vi "SPI_Example_Port Code_kyles_new_SM.vi"(11 "FPGA IO":T1={"SCLK"="DIO18", "CS_1"="DIO16", "MOSI"="DIO26", "MISO"="DIO25"}) -> ()   [LabVIEW 2012]
uses:
  Controls/FPGA SPI_Port Loop State.ctl
  <vilib>/rvi/DataTransferAndStorage/Container/Common/niFpgaContainerMetaDataKey.ctl
  <vilib>/rvi/DataTransferAndStorage/Container/Common/niFpgaContainerState.ctl
  <vilib>/rvi/DataTransferAndStorage/Container/Common/niFpgaDataTypeControl.ctl
  <vilib>/rvi/DataTransferAndStorage/Container/Common/niFpgaContainerImplementationControl.ctl
  <vilib>/rvi/DataTransferAndStorage/Container/Common/niFpgaContainerArbitrationOptionsControl.ctl
  <vilib>/rvi/DataTransferAndStorage/Container/Common/niFpgaTransferTypeControl.ctl
  <vilib>/rvi/DataTransferAndStorage/Container/Common/niFpgaContainerInitializationParameters.ctl
  <vilib>/rvi/Memory/Memory_Types/niFpgaMemoryInterfaceConfiguration.ctl
  <vilib>/rvi/FIFO/Fifo_Types/niFpgaFifoControlLogicControl.ctl
  Controls/FPGA SPI_SPI Loop State.ctl
  <vilib>/rvi/DataTransferAndStorage/Container/Common/niFpgaContainerGetUniqueNameForEmu.vi
  <vilib>/rvi/DataTransferAndStorage/Container/Common/niFpgaContainerSetEmuInfo.vi
  <vilib>/rvi/eio/common/nirviEmuReportErrorAndStop.vi
  Code/FPGA SPI_Globals.vi
  <vilib>/rvi/Emulation/niFpgaSctlEmulationGetInTimedLoop.vi
  <vilib>/rvi/Emulation/niFpgaSctlEmulationGlobalWrite.vi
  <vilib>/rvi/FIFO/Fifo_Resource/nirvififoEmulationSetSize.vi
  <vilib>/rvi/Emulation/niFpgaSctlEmulationFifoFullMgr.vi
  <vilib>/rvi/errors/niFpgaSetErrorForExecOnDevCompSimple.vi
  <vilib>/rvi/Emulation/niFpgaSctlEmulationResourceMgr.vi
  <vilib>/rvi/eio/common/nirviEmuTemplateMethod_errors.vi
  <vilib>/rvi/LocalResourceManager/LocalResourceManager.xnode
  <vilib>/rvi/DataTransferAndStorage/Container/XNode/niFpgaContainer.xnode
  <vilib>/rvi/FIFO/Fifo_Resource/nirvififoEmulationRead.vi
  <vilib>/rvi/FIFO/Fifo_Resource/nirvififoEmulationWrite.vi
  <vilib>/eio/EIONode/EIONode.xnode
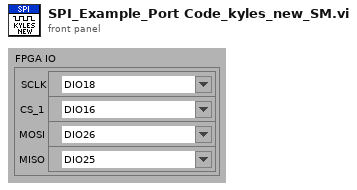
[diagram p1: front panel]
types:
  T1 = cluster{"SCLK":refnum<k21>, "CS_1":refnum<k21>, "MOSI":refnum<k21>, "MISO":refnum<k21>}
  T2 = typedef "FPGA SPI_Port Loop State.ctl" = enum8{"Idle", "Start", "Configure Hardware", "Start Hardware", "Set Done", "Wait Until Done", "Restart Port"}
  T3 = typedef "FPGA SPI_SPI Loop State.ctl" = enum8{"Initialize", "Set CS", "Read From FIFO", "Send Byte", "Write to FIFO", "Reset CS", "Read Delay"}
  T4 = typedef "FPGA SPI_Cmd.ctl" = enum8{"Idle", "Write/Read SPI", "Configure", "Restart"}
  T5 = cluster{"MOSI":bool[], "MISO":bool[], "Read?":bool}
  T6 = cluster{"Next State":T3, "Total Bytes":u16, "Future State":T3, "Read Wait":u32, "CS Reset Wait":u32, "Byte Count":u16}
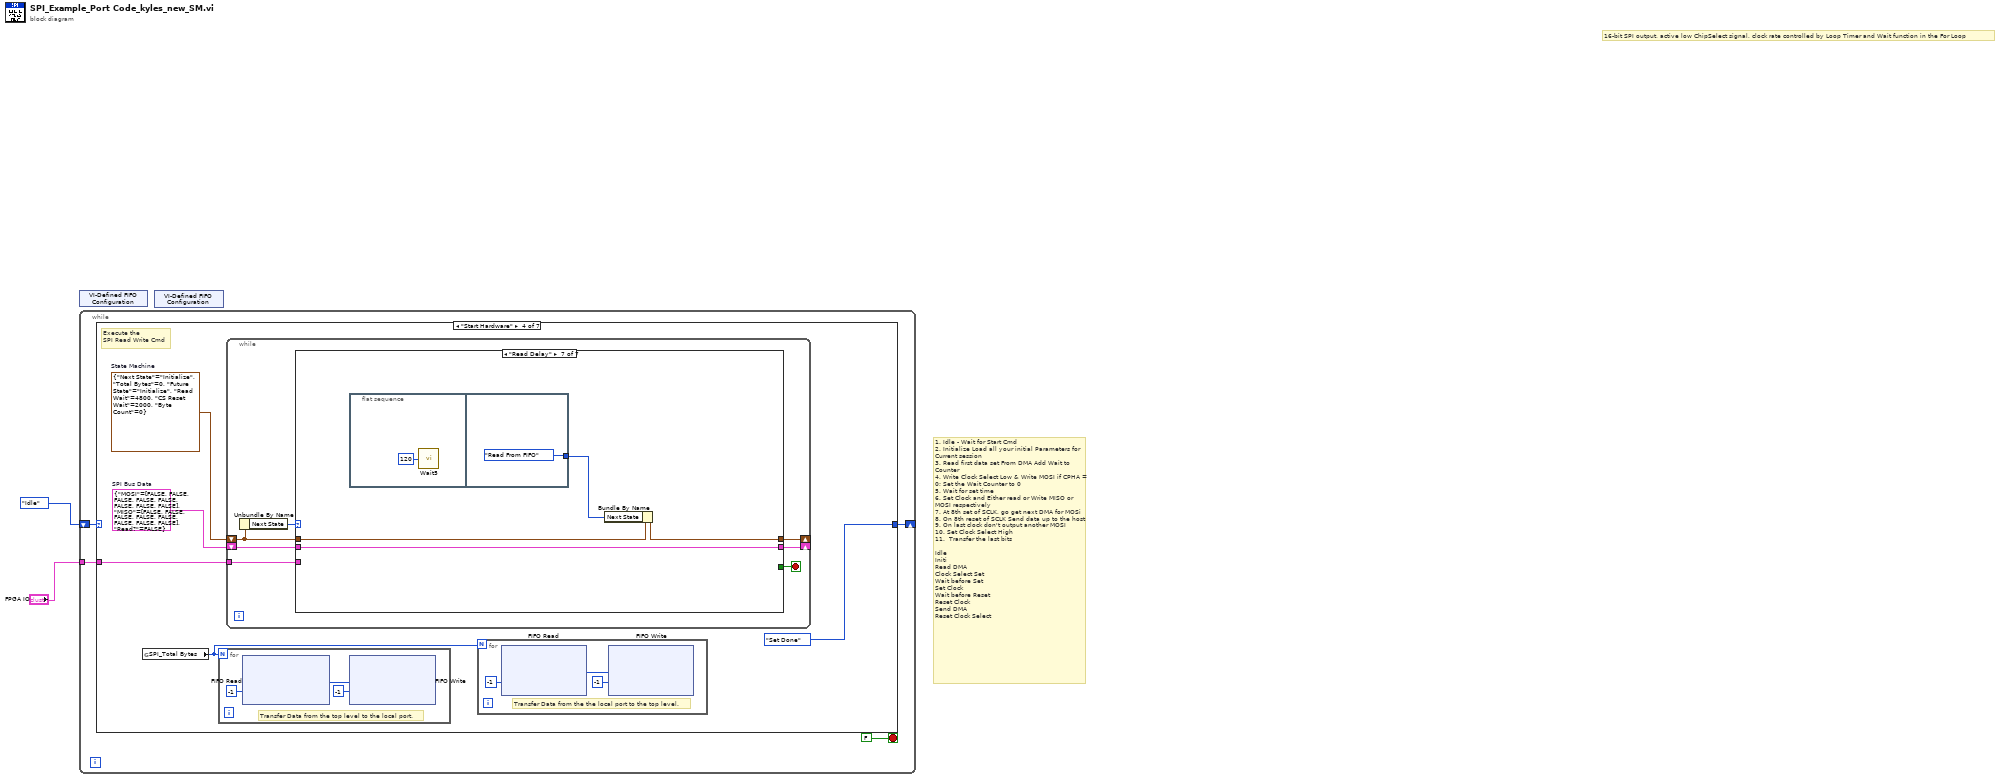
[diagram p0: block diagram]
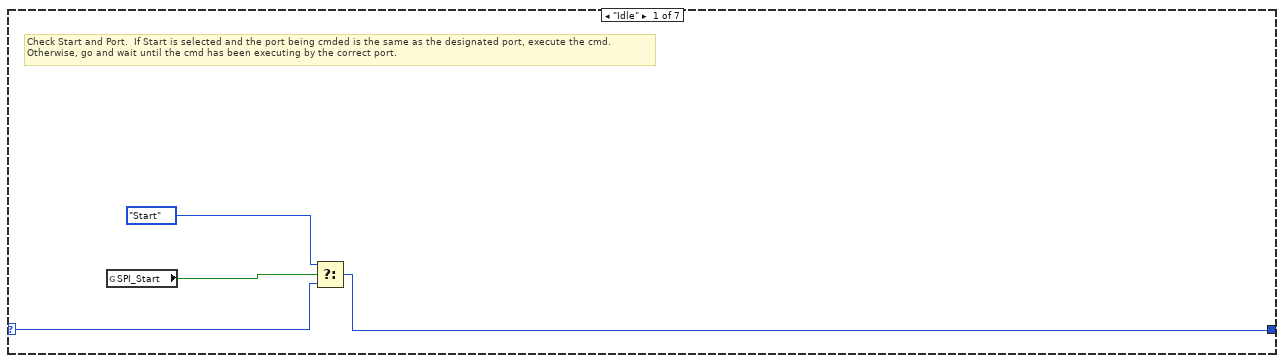
[diagram p2: hidden frame]
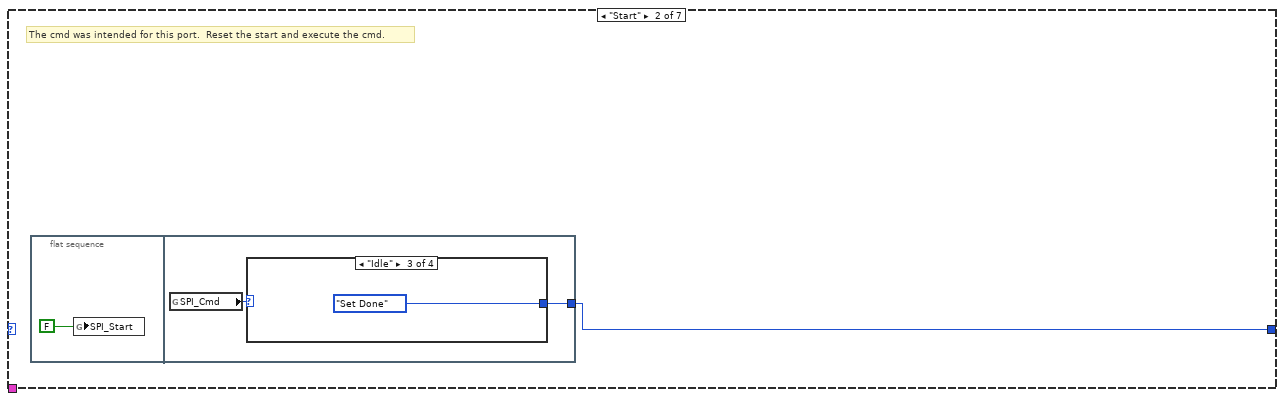
[diagram p3: hidden frame]
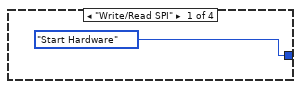
[diagram p4: hidden frame]
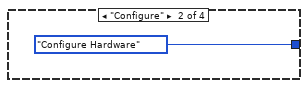
[diagram p5: hidden frame]
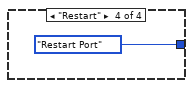
[diagram p6: hidden frame]
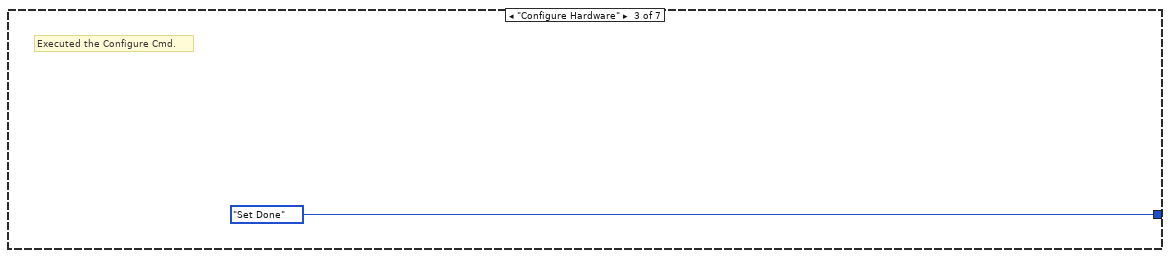
[diagram p7: hidden frame]
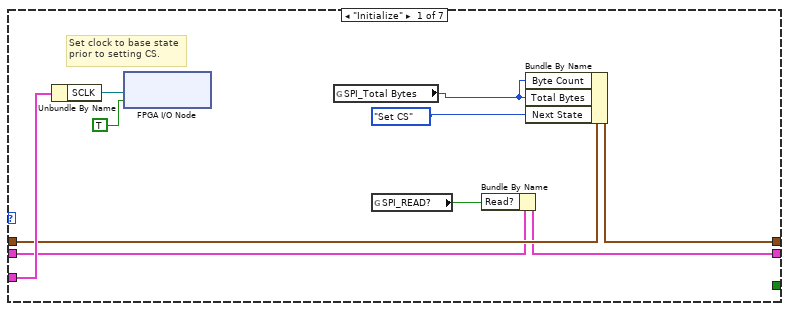
[diagram p8: hidden frame]
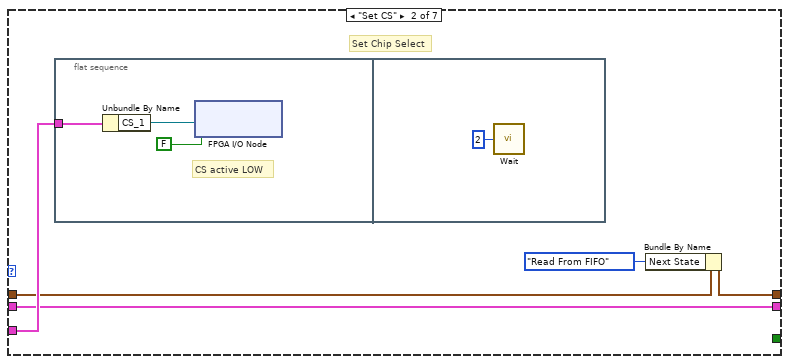
[diagram p9: hidden frame]
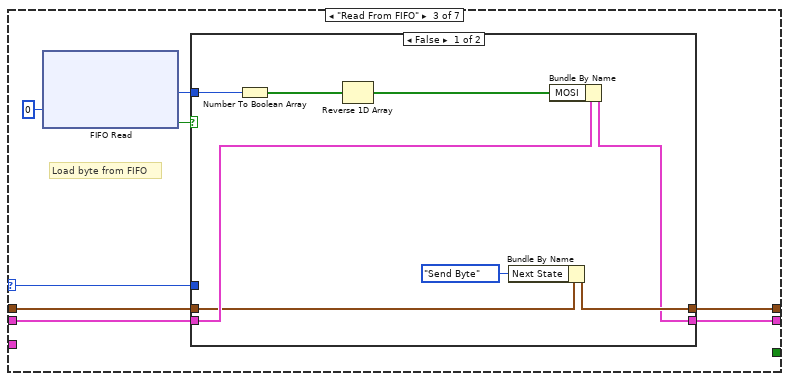
[diagram p10: hidden frame]
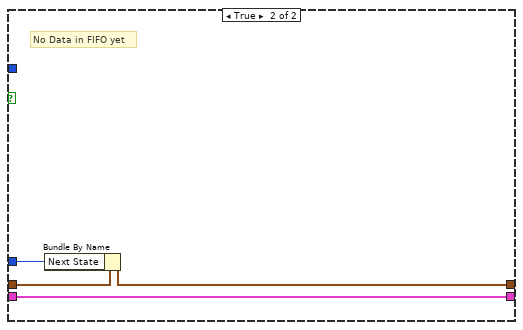
[diagram p11: hidden frame]
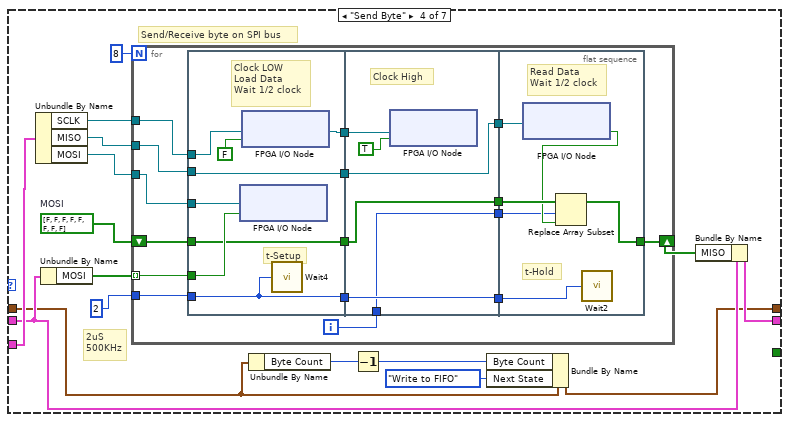
[diagram p12: hidden frame]
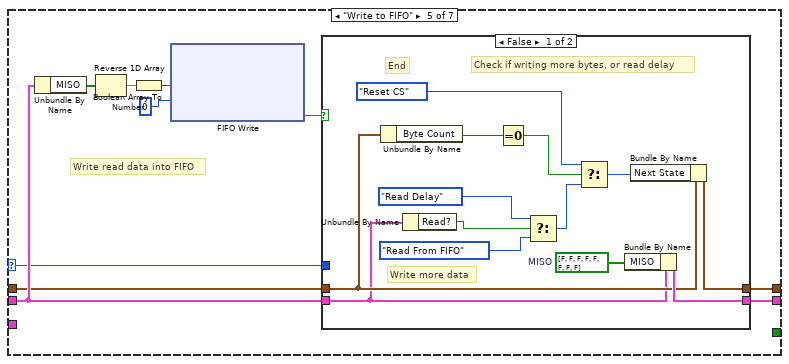
[diagram p13: hidden frame]
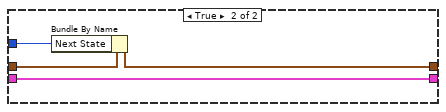
[diagram p14: hidden frame]
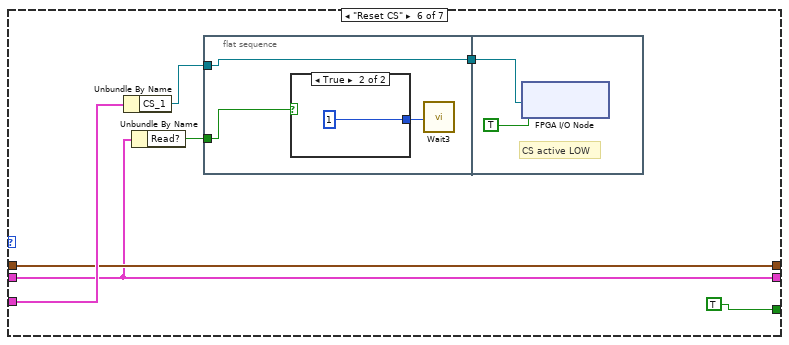
[diagram p15: hidden frame]
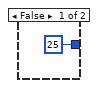
[diagram p16: hidden frame]
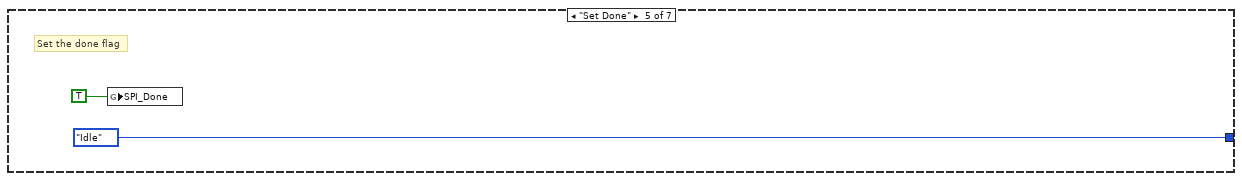
[diagram p17: hidden frame]
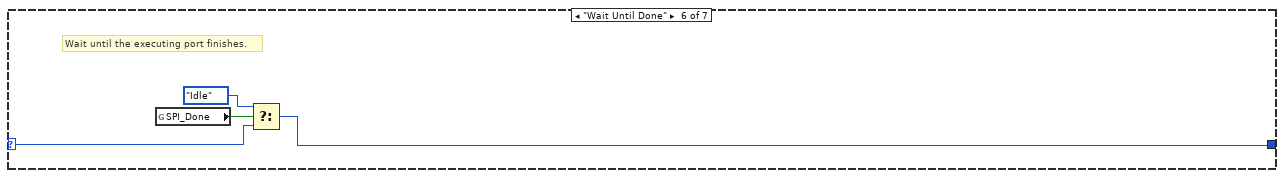
[diagram p18: hidden frame]
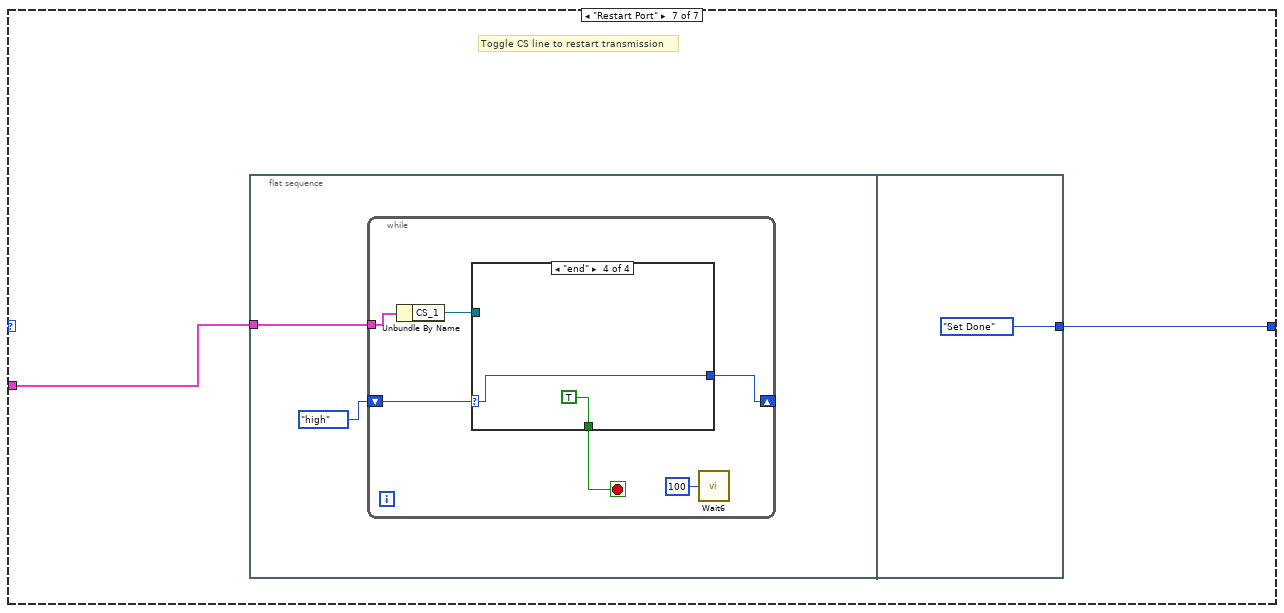
[diagram p19: hidden frame]
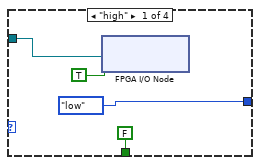
[diagram p20: hidden frame]
diagram:
  # "16-bit SPI output, active low ChipSelect signal, clock rate controlled by Loop Timer and Wait function in the For Loop"
  # "1. Idle - Wait for Start Cmd\n2. Initialize Load all your initial Parameters for Current session\n3. Read first data set From DMA Add Wait to Counter\n4. Write Clock Select Low & Write MOSI if CPHA = 0; Set the Wait Counter to 0\n5. Wait for set time\n6. Set Clock and Either read or Write MISO or MOSI respectively\n7. At 8th set of SCLK, go get next DMA for MOSi\n8. On 8th reset of SCLK Send data up to the host\n9. On last clock don't output another MOSI\n10. Set Clock Select High \n11.  Transfer the last bits\n\nIdle\nIniti\nRead DMA\nClock Select Set\nWait before Set\nSet Clock\nWait before Reset\nReset Clock\nSend DMA\nReset Clock Select"
  n1 = xnode "VI-Defined FIFO Configuration"() -> ()  [unwired: 1 out]
  n2 = while {
    shift-right: [w5] -> _
    shift-left: FPGA_SPI_Port_Loop_State."Idle" ("Action") -> [w4]
    tunnel: "FPGA IO" -> [w3]
    stop <- FALSE stop-if-true
    n3 = case shown="\"Start Hardware\"" w4 {
      selector: w4 -> [w7 _ _ _ _ w179 _]
      tunnel: [w9 w11 FPGA_SPI_Port_Loop_State."Set Done" ("Action") FPGA_SPI_Port_Loop_State."Set Done" ("Action") FPGA_SPI_Port_Loop_State."Idle" ("Action") w178 w182] -> w5
      tunnel: w3 -> [_ _ _ w23 _ _ w183]
      frame "Idle" {
        # "Check Start and Port.  If Start is selected and the port being cmded is the same as the designated port, execute the cmd.\nOtherwise, go and wait until the cmd has been executing by the correct port."
        n4 = global read "FPGA SPI_Globals.vi" "SPI_Start"() -> (w8:bool)
        n5 = Select(t=FPGA_SPI_Port_Loop_State."Start" ("Action"), s=w8, f=w7) -> (s? t:f=w9:T2)
      }
      frame "Start" {
        # "The cmd was intended for this port.  Reset the start and execute the cmd."
        n6 = flat-sequence {
          tunnel: [w13] -> w11
          frame #0 {
            n7 = global write "FPGA SPI_Globals.vi" "SPI_Start"(FALSE ("Write Flag")) -> ()
          }
          frame #1 {
            n8 = global read "FPGA SPI_Globals.vi" "SPI_Cmd"() -> (w14:T4)
            n9 = case shown="\"Idle\"" w14 {
              tunnel: [FPGA_SPI_Port_Loop_State."Start Hardware" ("Action") FPGA_SPI_Port_Loop_State."Configure Hardware" ("Action") FPGA_SPI_Port_Loop_State."Set Done" ("Action") FPGA_SPI_Port_Loop_State."Restart Port" ("Action")] -> w13
              frame "Write/Read SPI" {
              }
              frame "Configure" {
              }
              frame "Idle" {
              }
              frame "Restart" {
              }
            }
          }
        }
      }
      frame "Configure Hardware" {
        # "Executed the Configure Cmd."
      }
      frame "Start Hardware" {
        w21 = T5 {"MOSI"=[FALSE, FALSE, FALSE, FALSE, FALSE, FALSE, FALSE, FALSE], "MISO"=[FALSE, FALSE, FALSE, FALSE, FALSE, FALSE, FALSE, FALSE], "Read?"=FALSE}  # SPI Bus Data
        w22 = T6 {"Next State"=enum."Initialize", "Total Bytes"=0, "Future State"=enum."Initialize", "Read Wait"=4800, "CS Reset Wait"=2000, "Byte Count"=0}  # State Machine
        # "Execute the \nSPI Read Write Cmd"
        n10 = global read "FPGA SPI_Globals.vi" "SPI_Total Bytes"() -> (w20:u16)
        n11 = for {
          N: w20 -> [_]
          # "Transfer Data from the top level to the local port."
          n12 = xnode ("FIFO Read")("Timeout"=-1) -> ("Element"=w174:u8)  [unwired: 1 in, 2 out]
          n13 = xnode ("FIFO Write")("Element"=w174, "Timeout"=-1) -> ()  [unwired: 1 in, 2 out]
        }
        n14 = while {
          shift-right: [w31] -> _
          shift-left: w22 -> [w30]
          shift-right: [w27] -> _
          shift-left: w21 -> [w28]
          tunnel: w23 -> [w26]
          stop <- w25 stop-if-true
          n15 = Unbundle By Name(w30) -> ("Next State"=w29:T3)
          n16 = case shown="\"Read Delay\"" w29 {
            selector: w29 -> [_ _ w51 _ w125 _ _]
            tunnel: w30 -> [w39 w44 w53 w71 w124 w153 w167]
            tunnel: [w38 w46 w56 w79 w130 w153 w165] -> w31
            tunnel: w28 -> [w35 w43 w54 w81 w128 w151 w166]
            tunnel: [w33 w43 w55 w80 w127 w151 w166] -> w27
            tunnel: w26 -> [w41 w45 _ w86 _ w156 _]
            tunnel: [_ _ _ _ _ TRUE _] -> w25
            frame "Initialize" {
              # "Set clock to base state\nprior to setting CS."
              n17 = Unbundle By Name(w41) -> ("SCLK"=w40:refnum<k21>)
              n18 = xnode "FPGA I/O Node"("I/O Item"=TRUE, "FPGA I/O In"=w40) -> ()  [unwired: 1 out]
              n19 = global read "FPGA SPI_Globals.vi" "SPI_Total Bytes"() -> (w32:u16)
              n20 = global read "FPGA SPI_Globals.vi" "SPI_READ?"() -> (w36:bool)
              n21 = Bundle By Name(cluster=w35, "Read?"=w36) -> (w33:T5)
              n22 = Bundle By Name(cluster=w39, "Byte Count"=w32, "Total Bytes"=w32, "Next State"=FPGA_SPI_SPI_Loop_State."Set CS") -> (w38:T6)
            }
            frame "Set CS" {
              # "Set Chip Select"
              n23 = flat-sequence {
                tunnel: w45 -> [w49]
                frame #0 {
                  # "CS active LOW"
                  n24 = Unbundle By Name(w49) -> ("CS_1"=w48:refnum<k21>)
                  n25 = xnode "FPGA I/O Node"("I/O Item"=FALSE, "FPGA I/O In"=w48) -> ()  [unwired: 1 out]
                }
                frame #1 {
                  n26 = call "Wait"("Count(uSec)"=u8 2) -> ()  [unwired: 1 out]
                }
              }
              n27 = Bundle By Name(cluster=w44, "Next State"=FPGA_SPI_SPI_Loop_State."Read From FIFO") -> (w46:T6)
            }
            frame "Read From FIFO" {
              # "Load byte from FIFO"
              n28 = xnode ("FIFO Read")("Timeout"=0) -> ("Element"=w57:u8, "Timed Out?"=w52:bool)  [unwired: 1 in, 1 out]
              n29 = case shown="False" w52 {
                tunnel: w57 -> [w66 _]
                tunnel: [w65 w67] -> w56
                tunnel: [w64 w70] -> w55
                tunnel: w54 -> [w63 w70]
                tunnel: w53 -> [w61 w68]
                tunnel: w51 -> [_ w69]
                frame False {
                  n30 = Number To Boolean Array(number=w66) -> (Boolean array=w62:bool[])
                  n31 = Reverse 1D Array(array=w62) -> (reversed array=w59:bool[])
                  n32 = Bundle By Name(cluster=w61, "Next State"=FPGA_SPI_SPI_Loop_State."Send Byte") -> (w65:T6)
                  n33 = Bundle By Name(cluster=w63, "MOSI"=w59) -> (w64:T5)
                }
                frame True {
                  # "No Data in FIFO yet"
                  n34 = Bundle By Name(cluster=w68, "Next State"=w69) -> (w67:T6)
                }
              }
            }
            frame "Send Byte" {
              w76 = bool[] [FALSE, FALSE, FALSE, FALSE, FALSE, FALSE, FALSE, FALSE]  # MOSI
              # "2uS\n500KHz"
              # "Send/Receive byte on SPI bus"
              n35 = Unbundle By Name(w86) -> ("SCLK"=w85:refnum<k21>, "MISO"=w83:refnum<k21>, "MOSI"=w84:refnum<k21>)
              n36 = Unbundle By Name(w81) -> ("MOSI"=w72:bool[])
              n37 = for {
                N: 8 -> [_]
                tunnel: w72 -> [w102] mode=indexing
                tunnel: w85 -> [w101]
                tunnel: w84 -> [w100]
                tunnel: w83 -> [w99]
                tunnel: u32 2 ("Count(Ticks)") -> [w96]
                shift-right: [w88] -> w75
                shift-left: w76 -> [w92]
                i -> [w91]
                n38 = flat-sequence {
                  tunnel: w102 -> [w107]
                  tunnel: w101 -> [w110]
                  tunnel: w100 -> [w108]
                  tunnel: w99 -> [w106]
                  tunnel: [w106] -> w98
                  tunnel: [w105] -> w97
                  tunnel: w96 -> [w103]
                  tunnel: [w103] -> w95
                  tunnel: [w104] -> w93
                  tunnel: w92 -> [w104]
                  tunnel: w98 -> [w113]
                  tunnel: w97 -> [w114]
                  tunnel: w95 -> [w116]
                  tunnel: [w116] -> w94
                  tunnel: w93 -> [w112]
                  tunnel: w91 -> [w111]
                  tunnel: [w113] -> w90
                  tunnel: [w112] -> w89
                  tunnel: [w111] -> w87
                  tunnel: w94 -> [w122]
                  tunnel: w90 -> [w121]
                  tunnel: w89 -> [w120]
                  tunnel: [w119] -> w88
                  tunnel: w87 -> [w117]
                  frame #0 {
                    # "t-Setup"
                    # "Clock LOW\nLoad Data\nWait 1/2 clock"
                    n39 = xnode "FPGA I/O Node"("I/O Item"=w107, "FPGA I/O In"=w108) -> ()  [unwired: 1 out]
                    n40 = xnode "FPGA I/O Node"("I/O Item"=FALSE, "FPGA I/O In"=w110) -> ("FPGA I/O Out"=w105:refnum<k21>)
                    n41 = call "Wait4"("Count(uSec)"=w103) -> ()  [unwired: 1 out]
                  }
                  frame #1 {
                    # "Clock High"
                    n42 = xnode "FPGA I/O Node"("I/O Item"=TRUE, "FPGA I/O In"=w114) -> ()  [unwired: 1 out]
                  }
                  frame #2 {
                    # "Read Data\nWait 1/2 clock"
                    # "t-Hold"
                    n43 = xnode "FPGA I/O Node"("FPGA I/O In"=w121) -> ("I/O Item"=w118:bool)  [unwired: 1 out]
                    n44 = Replace Array Subset(array=w120, new element=w118, index=w117) -> (w119:bool[])
                    n45 = call "Wait2"("Count(uSec)"=w122) -> ()  [unwired: 1 out]
                  }
                }
              }
              n46 = Unbundle By Name(w71) -> ("Byte Count"=w74:u16)
              n47 = Decrement(x=w74) -> (x-1=w73:u16)
              n48 = Bundle By Name(cluster=w71, "Byte Count"=w73, "Next State"=FPGA_SPI_SPI_Loop_State."Write to FIFO") -> (w79:T6)
              n49 = Bundle By Name(cluster=w81, "MISO"=w75) -> (w80:T5)
            }
            frame "Write to FIFO" {
              # "Write read data into FIFO"
              n50 = Unbundle By Name(w128) -> ("MISO"=w132:bool[])
              n51 = Reverse 1D Array(array=w132) -> (reversed array=w123:bool[])
              n52 = Boolean Array To Number(Boolean array=w123) -> (number=w131:u8)
              n53 = xnode ("FIFO Write")("Element"=w131, "Timeout"=0) -> ("Timed Out?"=w126:bool)  [unwired: 1 in, 1 out]
              n54 = case shown="False" w126 {
                tunnel: [w145 w147] -> w130
                tunnel: w124 -> [w139 w148]
                tunnel: w128 -> [w134 w149]
                tunnel: [w141 w149] -> w127
                tunnel: w125 -> [_ w146]
                frame False {
                  w142 = bool[] [FALSE, FALSE, FALSE, FALSE, FALSE, FALSE, FALSE, FALSE]  # MISO
                  # "Check if writing more bytes, or read delay"
                  # "Write more data"
                  # "End"
                  n55 = Unbundle By Name(w139) -> ("Byte Count"=w137:u16)
                  n56 = Unbundle By Name(w134) -> ("Read?"=w133:bool)
                  n57 = Equal To 0?(x=w137) -> (x = 0?=w138:bool)
                  n58 = Select(t=FPGA_SPI_SPI_Loop_State."Read Delay", s=w133, f=FPGA_SPI_SPI_Loop_State."Read From FIFO" ("Next State")) -> (s? t:f=w136:T3)
                  n59 = Select(t=FPGA_SPI_SPI_Loop_State."Reset CS" ("Next State"), s=w138, f=w136) -> (s? t:f=w143:T3)
                  n60 = Bundle By Name(cluster=w134, "MISO"=w142) -> (w141:T5)
                  n61 = Bundle By Name(cluster=w139, "Next State"=w143) -> (w145:T6)
                }
                frame True {
                  n62 = Bundle By Name(cluster=w148, "Next State"=w146) -> (w147:T6)
                }
              }
            }
            frame "Reset CS" {
              n63 = Unbundle By Name(w156) -> ("CS_1"=w154:refnum<k21>)
              n64 = Unbundle By Name(w151) -> ("Read?"=w150:bool)
              n65 = flat-sequence {
                tunnel: w154 -> [w159]
                tunnel: [w159] -> w152
                tunnel: w150 -> [w158]
                tunnel: w152 -> [w162]
                frame #0 {
                  n66 = case shown="True" w158 {
                    tunnel: [u8 25 ("Count(uSec)") u8 1 ("Count(uSec)")] -> w157
                    frame False {
                    }
                    frame True {
                    }
                  }
                  n67 = call "Wait3"("Count(uSec)"=w157) -> ()  [unwired: 1 out]
                }
                frame #1 {
                  # "CS active LOW"
                  n68 = xnode "FPGA I/O Node"("I/O Item"=TRUE, "FPGA I/O In"=w162) -> ()  [unwired: 1 out]
                }
              }
            }
            frame "Read Delay" {
              n69 = flat-sequence {
                tunnel: [FPGA_SPI_SPI_Loop_State."Read From FIFO" ("Next State")] -> w164
                frame #0 {
                  n70 = call "Wait5"("Count(uSec)"=u16 120) -> ()  [unwired: 1 out]
                }
                frame #1 {
                }
              }
              n71 = Bundle By Name(cluster=w167, "Next State"=w164) -> (w165:T6)
            }
          }
        }
        n72 = for {
          N: w20 -> [_]
          # "Transfer Data from the the local port to the top level."
          n73 = xnode ("FIFO Read")("Timeout"=-1) -> ("Element"=w171:u8)  [unwired: 1 in, 2 out]
          n74 = xnode ("FIFO Write")("Element"=w171, "Timeout"=-1) -> ()  [unwired: 1 in, 2 out]
        }
      }
      frame "Set Done" {
        # "Set the done flag"
        n75 = global write "FPGA SPI_Globals.vi" "SPI_Done"(TRUE ("Done")) -> ()
      }
      frame "Wait Until Done" {
        # "Wait until the executing port finishes."
        n76 = global read "FPGA SPI_Globals.vi" "SPI_Done"() -> (w181:bool)
        n77 = Select(t=FPGA_SPI_Port_Loop_State."Idle" ("Action"), s=w181, f=w179) -> (s? t:f=w178:T2)
      }
      frame "Restart Port" {
        # "Toggle CS line to restart transmission"
        n78 = flat-sequence {
          tunnel: w183 -> [w185]
          tunnel: [FPGA_SPI_Port_Loop_State."Set Done" ("Action")] -> w182
          frame #0 {
            n79 = while {
              tunnel: w185 -> [w191]
              shift-right: [w186] -> _
              shift-left: enum16{"high", "low", "high_2", "end"}."high" -> [w187]
              stop <- w189 stop-if-true
              n80 = Unbundle By Name(w191) -> ("CS_1"=w190:refnum<k21>)
              n81 = case shown="\"end\"" w187 {
                selector: w187 -> [_ _ _ w204]
                tunnel: w190 -> [w194 w198 w202 _]
                tunnel: [FALSE FALSE FALSE TRUE] -> w189
                tunnel: [enum16{"high", "low", "high_2", "end"}."low" enum16{"high", "low", "high_2", "end"}."high_2" enum16{"high", "low", "high_2", "end"}."end" w204] -> w186
                frame "high" {
                  n82 = xnode "FPGA I/O Node"("I/O Item"=TRUE, "FPGA I/O In"=w194) -> ()  [unwired: 1 out]
                }
                frame "low" {
                  (unwired) i16 10000
                  n83 = xnode "FPGA I/O Node"("I/O Item"=FALSE, "FPGA I/O In"=w198) -> ()  [unwired: 1 out]
                }
                frame "high_2" {
                  n84 = xnode "FPGA I/O Node"("I/O Item"=TRUE, "FPGA I/O In"=w202) -> ()  [unwired: 1 out]
                }
                frame "end" {
                }
              }
              n85 = call "Wait6"("Count(uSec)"=u8 100 ("Count(Ticks)")) -> ()  [unwired: 1 out]
            }
          }
          frame #1 {
          }
        }
      }
    }
  }
  n86 = xnode "VI-Defined FIFO Configuration"() -> ()  [unwired: 1 out]
